vi "Trigger_and_Record_20210525.vi"() -> ()   [LabVIEW 2017]
uses:
  <vilib>/DAQmx/read.llb/DAQmx Read (Analog 1D Wfm NChan 1Samp).vi
  8b36a1b7-3159-42aa-b862-07ffc975086e.vi
  0fb37d18-2455-4527-a2db-066f6f4b2f85.vi
  <vilib>/DAQmx/write.llb/DAQmx Write (Digital Bool 1Line 1Point).vi
  <vilib>/DAQmx/write.llb/DAQmx Write (Analog DBL 1Chan 1Samp).vi
  <vilib>/DAQmx/write.llb/DAQmx Write (Analog Wfm 1Chan NSamp).vi
  <vilib>/DAQmx/create/channels.llb/DAQmx Create Channel (AO-Voltage-Basic).vi
  <vilib>/DAQmx/create/channels.llb/DAQmx Create Channel (AI-Voltage-Basic).vi
  <vilib>/DAQmx/create/channels.llb/DAQmx Create Channel (DO-Digital Output).vi
  <vilib>/DAQmx/miscellaneous.llb/DAQmx Fill In Error Info.vi
  <vilib>/DAQmx/configure/timing.llb/DAQmx Timing (Sample Clock).vi
  <vilib>/measure/NI_MABase.lvlib
panel:
  out "Current file name":path=path "C:/Users/Fukunaga/Documents/Xiaochen/Code/DMD_ephys/DataBackup/210509202912Ref.csv"
  out "Measurement 2":waveform(dbl)(graph)={"t0"=timestamp(0 s since 1904-01-01), "dt"=0.001, "Y"=[4.0, 4.0, 4.0, 4.0, 4.0, 4.0, 4.0, 4.0, 4.0, 4.0, 0.0, 0.0, 0.0, 0.0, 0.0, 0.0, 0.0, 0.0, 0.0, 0.0, 0.0, 0.0, 0.0, 0.0, 0.0, 0.0, 0.0, 0.0, 0.0, 0.0, 0.0, 0.0, 0.0, 0.0, 0.0, 0.0, 0.0, 0.0, 0.0, 0.0, 0.0, 0.0, 0.0, 0.0, 0.0, 0.0, 0.0, 0.0, 0.0, 0.0, 0.0, 0.0, 0.0, 0.0, 0.0, 0.0, 0.0, 0.0, 0.0, 0.0, 0.0, 0.0, 0.0, 0.0, 0.0, 0.0, 0.0, 0.0, 0.0, 0.0, 0.0, 0.0, 0.0, 0.0, 0.0, 0.0, 0.0, 0.0, 0.0, 0.0, 0.0, 0.0, 0.0, 0.0, 0.0, 0.0, 0.0, 0.0, 0.0, 0.0, 0.0, 0.0, 0.0, 0.0, 0.0, 0.0, 0.0, 0.0, 0.0, 0.0, 4.0, 4.0, 4.0, 4.0, 4.0, 4.0, 4.0, 4.0, 4.0, 4.0, 0.0, 0.0, 0.0, 0.0, 0.0, 0.0, 0.0, 0.0, 0.0, 0.0, 0.0, 0.0, 0.0, 0.0, 0.0, 0.0, 0.0, 0.0, 0.0, 0.0, 0.0, 0.0, 0.0, 0.0, 0.0, 0.0, 0.0, 0.0, 0.0, 0.0, 0.0, 0.0, 0.0, 0.0, 0.0, 0.0, 0.0, 0.0, 0.0, 0.0, 0.0, 0.0, 0.0, 0.0, 0.0, 0.0, 0.0, 0.0, 0.0, 0.0, 0.0, 0.0, 0.0, 0.0, 0.0, 0.0, 0.0, 0.0, 0.0, 0.0, 0.0, 0.0, 0.0, 0.0, 0.0, 0.0, 0.0, 0.0, 0.0, 0.0, 0.0, 0.0, 0.0, 0.0, 0.0, 0.0, 0.0, 0.0, 0.0, 0.0, 0.0, 0.0, 0.0, 0.0, 0.0, 0.0, 0.0, 0.0, 0.0, 0.0, 4.0, 4.0, 4.0, 4.0, 4.0, 4.0, 4.0, 4.0, 4.0, 4.0, 0.0, 0.0, 0.0, 0.0, 0.0, 0.0, 0.0, 0.0, 0.0, 0.0, 0.0, 0.0, 0.0, 0.0, 0.0, 0.0, 0.0, 0.0, 0.0, 0.0, 0.0, 0.0, 0.0, 0.0, 0.0, 0.0, 0.0, 0.0, 0.0, 0.0, 0.0, 0.0, 0.0, 0.0, 0.0, 0.0, 0.0, 0.0, 0.0, 0.0, 0.0, 0.0, 0.0, 0.0, 0.0, 0.0, 0.0, 0.0, 0.0, 0.0, 0.0, 0.0, 0.0, 0.0, 0.0, 0.0, 0.0, 0.0, 0.0, 0.0, 0.0, 0.0, 0.0, 0.0, 0.0, 0.0, 0.0, 0.0, 0.0, 0.0, 0.0, 0.0, 0.0, 0.0, 0.0, 0.0, 0.0, 0.0, 0.0, 0.0, 0.0, 0.0, 0.0, 0.0, 0.0, 0.0, 0.0, 0.0, 0.0, 0.0]} caption="output_ Analog"
  out "LED Driver":waveform(dbl)(graph)={"t0"=timestamp(3703404563.058236 s since 1904-01-01), "dt"=0.001, "Y"=[0.0005036777732009539], "attributes"=variant("NI_ChannelName"=variant(string "Dev1/ai4"), "NI_UnitDescription"=variant(string "Volts"))}
  out "Optometer misc":waveform(dbl)(graph)={"t0"=timestamp(3703404563.058236 s since 1904-01-01), "dt"=0.001, "Y"=[-0.01620720196889872], "attributes"=variant("NI_ChannelName"=variant(string "Dev1/ai0"), "NI_UnitDescription"=variant(string "Volts"))} caption="Optometer  MISC"
  in  "Wait for display (ms)":u32=400
  in  "Result path":path=path "C:/Users/Fukunaga/Documents/Xiaochen/Code/DMD_ephys/DataBackup"
  in  "Sample rate":dbl=1000.0 format="%0.2f"
  in  "DO Upload DMD":tag="Dev1/port1/line1"
  in  "Combo Box":string(combo)="LaserDiode"
  in  "Driving Current\nAmplitude (mA)":dbl=400.0 format="%0.2f"
  in  "AO Illumination":tag="Dev1/ao0"
  in  "time for uploading (ms)":u32=2200
  in  "Number of Pulse":i8=1
  in  "DMD Pulse \nDuration (ms)":dbl=240.0
  in  "Frequency of Pulse (Hz)":dbl=3.0
  in  "AO Trigger DMD":tag="Dev1/ao1"
  in  "Stop Sampling":bool
  in  "latency between two stimuli":u32=1000
  in  "Stop Stimuli":bool
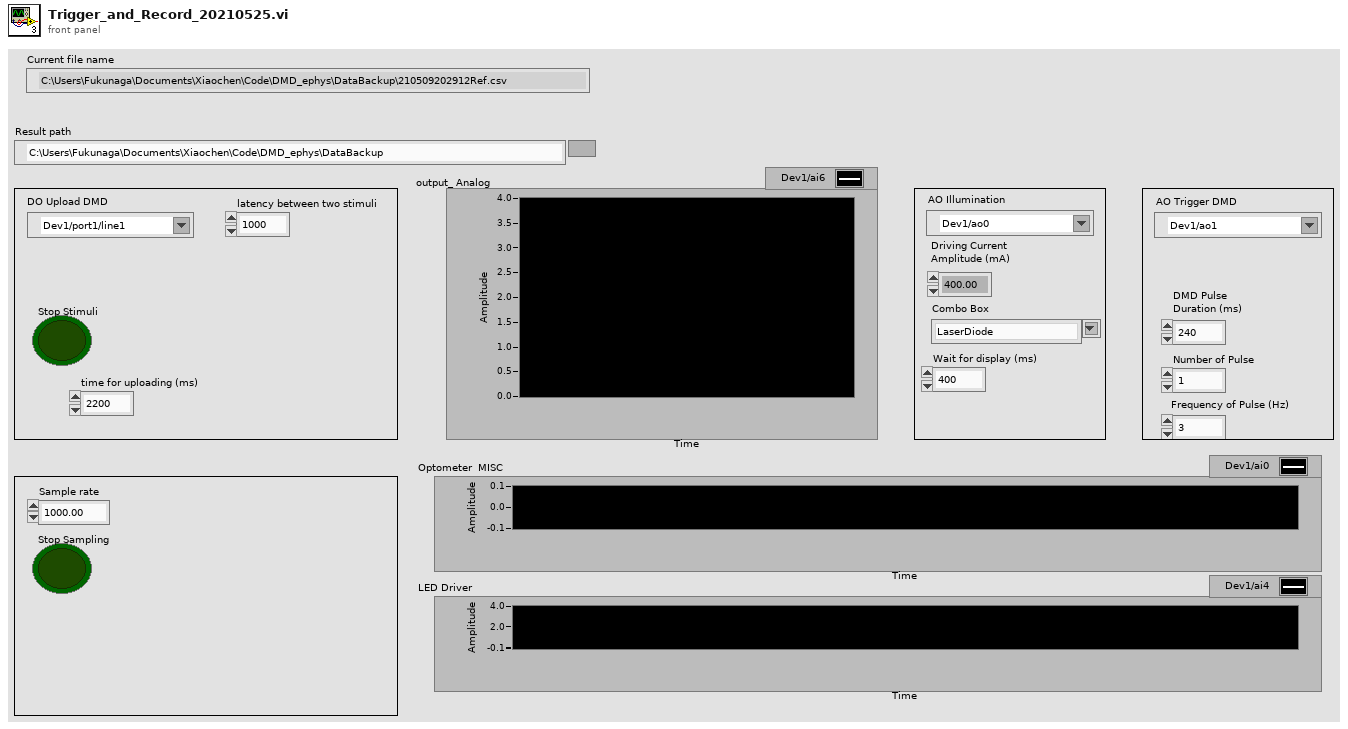
[diagram p1: front panel]
types:
  T1 = enum16{"open", "replace", "create", "open or create", "replace or create", "replace or create with confirmation"}
  T2 = enum16{"Sine Wave", "Triangle Wave", "Square Wave", "Sawtooth Wave"}
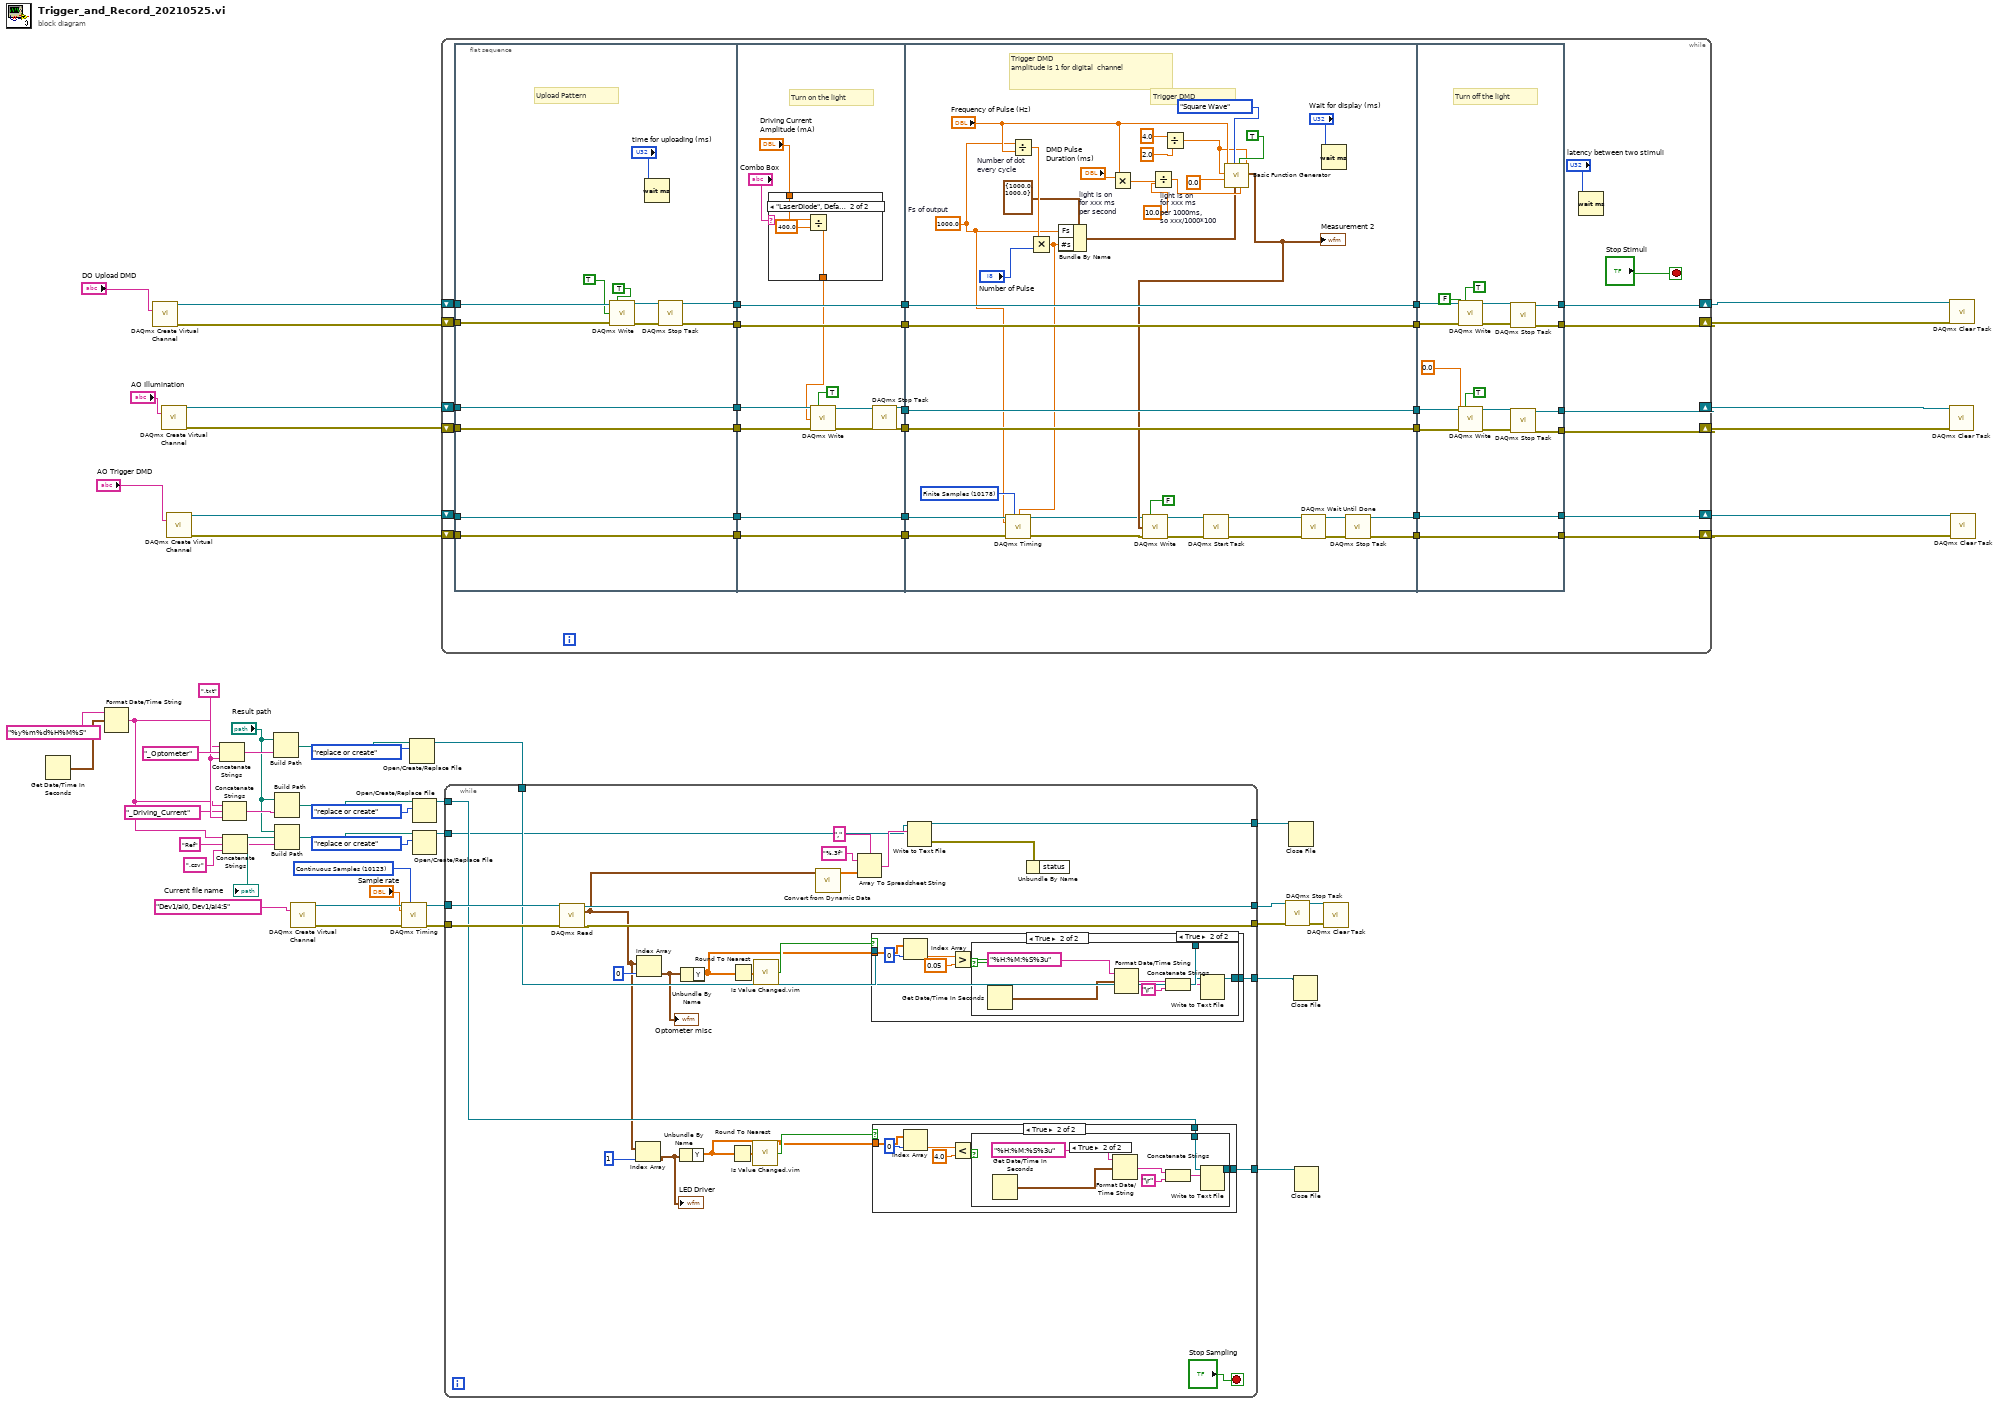
[diagram p0: block diagram]
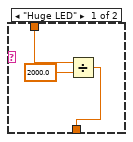
[diagram p6: hidden frame]
diagram:
  w7 = ".txt" ("string")
  w13 = 10123 items=["Finite Samples"=10178, "Continuous Samples"=10123, "Hardware Timed Single Point"=12522] ("sample mode")
  n1 = Get Date/Time In Seconds() -> (seconds since 1Jan1904=w11:timestamp)
  n2 = Format Date/Time String(time format string (%c)="%y%m%d%H%M%S", seconds (now)=w11) -> (date/time string=w5:string)  [unwired: 1 in]
  n3 = call-poly <vilib>:"DAQmx Create Virtual Channel.vi"("lines"="DO Upload DMD") -> ("task out"=w50:refnum<k21>, "error out"=w49:errorcluster)  [unwired: 13 in]
  n4 = call-poly <vilib>:"DAQmx Create Virtual Channel.vi"("physical channels"="AO Illumination") -> ("task out"=w45:refnum<k21>, "error out"=w47:errorcluster)  [unwired: 13 in]
  n5 = call-poly <vilib>:"DAQmx Create Virtual Channel.vi"("physical channels"="AO Trigger DMD") -> ("task out"=w17:refnum<k21>, "error out"=w38:errorcluster)  [unwired: 13 in]
  n6 = Concatenate Strings(w5, "_Optometer" ("string"), w7) -> (w4:string)
  n7 = Concatenate Strings(w5, "_Driving_Current" ("string"), w7) -> (w3:string)
  n8 = Concatenate Strings(w5, "Ref" ("string"), ".csv" ("string")) -> (w2:string)
  n9 = Build Path(base path="Result path", name or relative path=w4) -> (appended path=w26:path)
  n10 = Build Path(base path="Result path", name or relative path=w3) -> (appended path=w25:path)
  n11 = Build Path(base path="Result path", name or relative path=w2) -> (appended path=w21:path)
  "Current file name" <- w21
  n12 = call-poly <vilib>:"DAQmx Create Virtual Channel.vi"("physical channels"=tag "Dev1/ai0, Dev1/ai4:5" ("Input channel 1")) -> ("task out"=w32:refnum<k21>, "error out"=w33:errorcluster)  [unwired: 13 in]
  n13 = call-poly <vilib>:"DAQmx Timing.vi"("task/channels in"=w32, "sample mode"=w13, "rate"="Sample rate", "error in"=w33) -> ("task out"=w31:refnum<k21>, "error out"=w34:errorcluster)  [unwired: 10 in]
  n14 = Open/Create/Replace File(file path (use dialog)=w26, operation (0:open)=T1."replace or create") -> (refnum out=w23:refnum<file>)  [unwired: 4 in, 2 out]
  n15 = Open/Create/Replace File(file path (use dialog)=w25, operation (0:open)=T1."replace or create") -> (refnum out=w22:refnum<file>)  [unwired: 4 in, 2 out]
  n16 = Open/Create/Replace File(file path (use dialog)=w21, operation (0:open)=T1."replace or create") -> (refnum out=w19:refnum<file>)  [unwired: 4 in, 2 out]
  n17 = while {
    shift-right: [w80] -> w14
    shift-left: w50 -> [w81]
    shift-right: [w78] -> w48
    shift-left: w49 -> [w79]
    shift-right: [w62] -> w46
    shift-left: w47 -> [w74]
    shift-right: [w61] -> w36
    shift-left: w45 -> [w72]
    shift-right: [w56] -> w35
    shift-left: w17 -> [w60]
    shift-right: [w54] -> w37
    shift-left: w38 -> [w51]
    stop <- "Stop Stimuli" stop-if-true
    n18 = flat-sequence {
      tunnel: w81 -> [w92]
      tunnel: w79 -> [w90]
      tunnel: [w91] -> w77
      tunnel: [w89] -> w76
      tunnel: w74 -> [w88]
      tunnel: [w88] -> w73
      tunnel: w72 -> [w84]
      tunnel: [w84] -> w71
      tunnel: w60 -> [w87]
      tunnel: [w87] -> w59
      tunnel: [w86] -> w52
      tunnel: w51 -> [w86]
      tunnel: w77 -> [w108]
      tunnel: w76 -> [w107]
      tunnel: w73 -> [w105]
      tunnel: w71 -> [w102]
      tunnel: [w108] -> w70
      tunnel: [w107] -> w69
      tunnel: [w105] -> w68
      tunnel: [w103] -> w67
      tunnel: w59 -> [w100]
      tunnel: [w100] -> w58
      tunnel: [w99] -> w53
      tunnel: w52 -> [w99]
      tunnel: w70 -> [w147]
      tunnel: w69 -> [w146]
      tunnel: w68 -> [w145]
      tunnel: w67 -> [w144]
      tunnel: [w147] -> w66
      tunnel: [w146] -> w65
      tunnel: [w145] -> w64
      tunnel: [w144] -> w63
      tunnel: w58 -> [w120]
      tunnel: [w115] -> w57
      tunnel: [w143] -> w55
      tunnel: w53 -> [w140]
      tunnel: [w149] -> w78
      tunnel: [w150] -> w80
      tunnel: w66 -> [w152]
      tunnel: w65 -> [w151]
      tunnel: w64 -> [w158]
      tunnel: w63 -> [w159]
      tunnel: [w161] -> w62
      tunnel: [w160] -> w61
      tunnel: w57 -> [w157]
      tunnel: [w157] -> w56
      tunnel: w55 -> [w156]
      tunnel: [w156] -> w54
      frame #0 {
        # "Upload Pattern"
        n19 = call-poly <vilib>:"DAQmx Write.vi"("task/channels in"=w92, "auto start"=TRUE, "data"=TRUE, "error in"=w90) -> ("task out"=w94:refnum<k21>, "error out"=w93:errorcluster)  [unwired: 9 in, 1 out]
        n20 = Wait (ms)(milliseconds to wait="time for uploading (ms)") -> ()  [unwired: 1 out]
        n21 = call <vilib>:"DAQmx Stop Task.vi"("task/channels in"=w94, "error in"=w93) -> ("task out"=w91:refnum<k21>, "error out"=w89:errorcluster)  [unwired: 12 in]
      }
      frame #1 {
        # "Turn on the light"
        n22 = case shown="\"LaserDiode\", Default" "Combo Box" {
          tunnel: "Driving Current\nAmplitude (mA)" -> [w111 w114]
          tunnel: [w109 w112] -> w97
          frame "Huge LED" {
            n23 = Divide(x=w111, y=2000.0) -> (x/y=w109:dbl)
          }
          frame "LaserDiode", Default {
            n24 = Divide(x=w114, y=400.0) -> (x/y=w112:dbl)
          }
        }
        n25 = call-poly <vilib>:"DAQmx Write.vi"("task/channels in"=w102, "auto start"=TRUE, "data"=w97, "error in"=w105) -> ("task out"=w104:refnum<k21>, "error out"=w106:errorcluster)  [unwired: 9 in, 1 out]
        n26 = call <vilib>:"DAQmx Stop Task.vi"("task/channels in"=w104, "error in"=w106) -> ("task out"=w103:refnum<k21>)  [unwired: 12 in, 1 out]
      }
      frame #2 {
        w118 = 10178 items=["Finite Samples"=10178, "Continuous Samples"=10123, "Hardware Timed Single Point"=12522] ("sample mode")
        w117 = 1000.0  # Fs of output
        # "Trigger DMD\namplitude is 1 for digital  channel"
        # "Trigger DMD"
        n27 = Divide "Number of dot \nevery cycle"(x=w117, y="Frequency of Pulse (Hz)") -> (x/y=w135:dbl)
        n28 = Multiply(x=w135, y="Number of Pulse") -> (x*y=w116:dbl)
        n29 = call-poly <vilib>:"DAQmx Timing.vi"("task/channels in"=w120, "sample mode"=w118, "samples per channel"=w116, "rate"=w117) -> ("task out"=w119:refnum<k21>)  [unwired: 10 in, 1 out]
        n30 = Bundle By Name(cluster=cluster{"Fs":dbl, "#s":dbl} {"Fs"=1000.0, "#s"=1000.0} ("sampling info"), "Fs"=w117, "#s"=w116) -> (w133:cluster{"Fs":dbl, "#s":dbl})
        n31 = Multiply "light is on \nfor xxx ms \nper second"(x="DMD Pulse \nDuration (ms)", y="Frequency of Pulse (Hz)") -> (x*y=w138:dbl)
        n32 = Divide "light is on \nfor xxx ms \nper 1000ms,\nso xxx/1000*100"(x=w138, y=10.0) -> (x/y=w139:dbl)
        n33 = Divide(x=4.0, y=2.0) -> (x/y=w123:dbl)
        n34 = call <vilib>:"Basic Function Generator.vi"("offset"=w123, "square wave duty cycle (%)"=w139, "reset signal"=TRUE, "sampling info"=w133, "signal type"=T2."Square Wave", "phase"=0.0, "amplitude"=w123, "frequency"="Frequency of Pulse (Hz)") -> ("signal out"=w126:waveform(dbl))  [unwired: 1 in, 2 out]
        "Measurement 2" <- w126
        n35 = call-poly <vilib>:"DAQmx Write.vi"("task/channels in"=w119, "auto start"=FALSE, "data"=w126, "error in"=w140) -> ("task out"=w142:refnum<k21>, "error out"=w143:errorcluster)  [unwired: 9 in, 1 out]
        n36 = call <vilib>:"DAQmx Start Task.vi"("task/channels in"=w142) -> ("task out"=w122:refnum<k21>)  [unwired: 13 in, 1 out]
        n37 = call <vilib>:"DAQmx Wait Until Done.vi"("task/channels in"=w122) -> ("task out"=w121:refnum<k21>)  [unwired: 13 in, 1 out]
        n38 = Wait (ms)(milliseconds to wait="Wait for display (ms)") -> ()  [unwired: 1 out]
        n39 = call <vilib>:"DAQmx Stop Task.vi"("task/channels in"=w121) -> ("task out"=w115:refnum<k21>)  [unwired: 13 in, 1 out]
      }
      frame #3 {
        # "Turn off the light"
        n40 = call-poly <vilib>:"DAQmx Write.vi"("task/channels in"=w152, "auto start"=TRUE, "data"=FALSE, "error in"=w151) -> ("task out"=w154:refnum<k21>, "error out"=w155:errorcluster)  [unwired: 9 in, 1 out]
        n41 = call-poly <vilib>:"DAQmx Write.vi"("task/channels in"=w159, "auto start"=TRUE, "data"=0.0 ("data 2"), "error in"=w158) -> ("task out"=w164:refnum<k21>, "error out"=w165:errorcluster)  [unwired: 9 in, 1 out]
        n42 = call <vilib>:"DAQmx Stop Task.vi"("task/channels in"=w154, "error in"=w155) -> ("task out"=w150:refnum<k21>, "error out"=w149:errorcluster)  [unwired: 12 in]
        n43 = call <vilib>:"DAQmx Stop Task.vi"("task/channels in"=w164, "error in"=w165) -> ("task out"=w160:refnum<k21>, "error out"=w161:errorcluster)  [unwired: 12 in]
      }
    }
    n44 = Wait (ms)(milliseconds to wait="latency between two stimuli") -> ()  [unwired: 1 out]
  }
  n45 = while {
    tunnel: w31 -> [w191]
    tunnel: w34 -> [w190]
    tunnel: [w189] -> w42
    tunnel: [w188] -> w41
    tunnel: [w183] -> w29
    tunnel: [w182] -> w28
    tunnel: w23 -> [w181]
    tunnel: w22 -> [w180]
    tunnel: w19 -> [w170]
    tunnel: [w169] -> w18
    stop <- "Stop Sampling" stop-if-true
    n46 = call-poly <vilib>:"DAQmx Read.vi"("task/channels in"=w191, "error in"=w190) -> ("task out"=w189:refnum<k21>, "data"=w166:waveform(dbl)[], "error out"=w188:errorcluster)  [unwired: 11 in]
    n47 = Index Array(array=w166, index=1) -> (element=w167:waveform(dbl))
    "LED Driver" <- w167
    n48 = Index Array(array=w166, index=0) -> (element=w168:waveform(dbl))
    "Optometer misc" <- w168
    n49 = Unbundle By Name(w167) -> ("Y"=w177:dbl[])
    n50 = Unbundle By Name(w168) -> ("Y"=w176:dbl[])
    n51 = Round To Nearest(number=w177) -> (nearest integer value=w184:dbl[])
    n52 = Round To Nearest(number=w176) -> (nearest integer value=w185:dbl[])
    n53 = call "Is Value Changed.vim"("value"=w184) -> ("changed or first call?"=w178:bool)
    n54 = call "Is Value Changed.vim"("value"=w185) -> ("changed or first call?"=w179:bool)
    n55 = call "Convert from Dynamic Data"("Dynamic Data Type"=w166) -> ("Array"=w171:dbl[][])  [unwired: 3 in]
    n56 = Array To Spreadsheet String(delimiter (Tab)=",", array=w171, 3:"%.3f" ("format string")) -> (spreadsheet string=w172:string)
    n57 = case shown="True" w179 {
      tunnel: [w209 w216] -> w183
      tunnel: w176 -> [_ w215]
      tunnel: w181 -> [w209 w210]
      frame False {
      }
      frame True {
        n58 = Index Array(array=w215, index=0) -> (element=w213:dbl)
        n59 = Greater?(x=w213, y=0.05) -> (0:w211:bool)
        n60 = case shown="True" w211 {
          tunnel: [w217 w224] -> w216
          tunnel: w210 -> [w217 w221]
          frame False {
          }
          frame True {
            n61 = Get Date/Time In Seconds() -> (seconds since 1Jan1904=w220:timestamp)
            n62 = Format Date/Time String(time format string (%c)="%H:%M:%S%3u", seconds (now)=w220) -> (date/time string=w219:string)  [unwired: 1 in]
            n63 = Concatenate Strings(w219, "\r") -> (w222:string)
            n64 = Write to Text File(file (use dialog)=w221, text=w222) -> (refnum out=w224:refnum<file>)  [unwired: 2 in, 2 out]
          }
        }
      }
    }
    n65 = case shown="True" w178 {
      tunnel: [w193 w200] -> w182
      tunnel: w177 -> [_ w199]
      tunnel: w180 -> [w193 w194]
      frame False {
      }
      frame True {
        n66 = Index Array(array=w199, index=0) -> (element=w197:dbl)
        n67 = Less?(x=w197, y=4.0) -> (x < y?=w195:bool)
        n68 = case shown="True" w195 {
          tunnel: [w201 w208] -> w200
          tunnel: w194 -> [w201 w205]
          frame False {
          }
          frame True {
            n69 = Get Date/Time In Seconds() -> (seconds since 1Jan1904=w204:timestamp)
            n70 = Format Date/Time String(time format string (%c)="%H:%M:%S%3u", seconds (now)=w204) -> (date/time string=w203:string)  [unwired: 1 in]
            n71 = Concatenate Strings(w203, "\r") -> (w206:string)
            n72 = Write to Text File(file (use dialog)=w205, text=w206) -> (refnum out=w208:refnum<file>)  [unwired: 2 in, 2 out]
          }
        }
      }
    }
    n73 = Write to Text File(file (use dialog)=w170, text=w172) -> (refnum out=w169:refnum<file>, error out=w175:errorcluster)  [unwired: 2 in, 1 out]
    n74 = Unbundle By Name(w175) -> ()  [unwired: 1 out]
  }
  n75 = call <vilib>:"DAQmx Stop Task.vi"("task/channels in"=w42, "error in"=w41) -> ("task out"=w40:refnum<k21>, "error out"=w39:errorcluster)  [unwired: 12 in]
  n76 = Close File(refnum=w18) -> ()  [unwired: 1 in, 2 out]
  n77 = Close File(refnum=w29) -> ()  [unwired: 1 in, 2 out]
  n78 = Close File(refnum=w28) -> ()  [unwired: 1 in, 2 out]
  n79 = call <vilib>:"DAQmx Clear Task.vi"("task in"=w40, "error in"=w39) -> ()  [unwired: 13 in, 1 out]
  n80 = call <vilib>:"DAQmx Clear Task.vi"("task in"=w36, "error in"=w46) -> ()  [unwired: 13 in, 1 out]
  n81 = call <vilib>:"DAQmx Clear Task.vi"("task in"=w14, "error in"=w48) -> ()  [unwired: 13 in, 1 out]
  n82 = call <vilib>:"DAQmx Clear Task.vi"("task in"=w35, "error in"=w37) -> ()  [unwired: 13 in, 1 out]
